vi "SetupConfiguration.vi"   [LabVIEW 2011]
panel:
  # "Configuration for setup in room D012, right side"
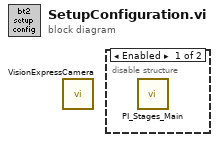
[diagram p0: block diagram]
diagram:
  n1 = call "VisionExpressCamera.vi"() -> ()  [unwired: 12 in]
  n2 = disable-structure shown="Enabled" {
    frame Enabled {
      n3 = call "PI_Stages_Main.vi"() -> ()  [unwired: 12 in]
    }
    frame Disabled {
    }
  }
